vi "Tc filter.vi"(6 "Reset":bool, 9 "Fs":dbl=1.0, 10 "Tc":dbl, 11 "Input":dbl) -> (3 "Output":dbl)   [LabVIEW 2014]
panel:
  # "Time constant of filter (Fs units)"
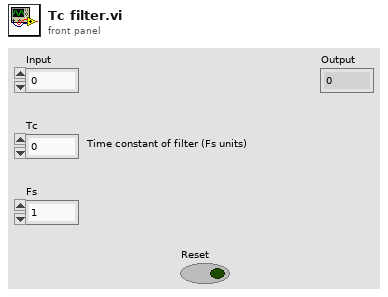
[diagram p1: front panel]
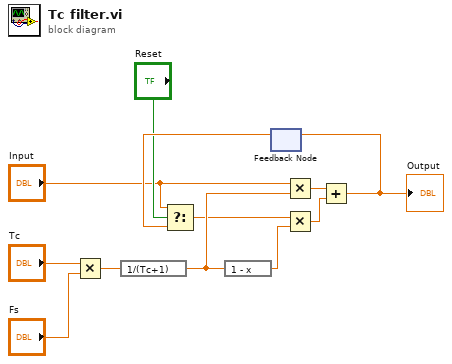
[diagram p0: block diagram]
diagram:
  n1 = Multiply(x="Tc", y="Fs") -> (x*y=w2:dbl)
  n2 = expression code="1/(Tc+1)"(w2) -> (w10:dbl)
  n3 = expression code="1 - x"(w10) -> (w9:dbl)
  n4 = feedback #1() -> (w6:dbl)  [unwired: 1 in]
  n5 = Select(t="Input", s="Reset", f=w6) -> (s? t:f=w7:dbl)
  n6 = Multiply(x="Input", y=w10) -> (x*y=w11:dbl)
  n7 = Multiply(x=w7, y=w9) -> (x*y=w12:dbl)
  n8 = Add(x=w11, y=w12) -> (x+y=w8:dbl)
  "Output" <- w8
  n9 = feedback-in #1(w8) -> ()
